vi "MCP2221_SetGpioSettings.vi"(8 "error in":errorcluster, 9 "handle in":i32, 10 "outputValues":u8[](array[numeric]), 11 "pinDirections":u8[](array[numeric])) -> (0 "error out":errorcluster, 1 "handle out":i32, 3 "return type":i32)   [LabVIEW 2025]
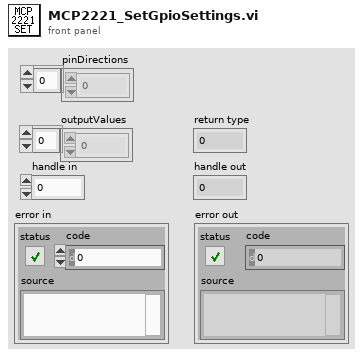
[diagram p1: front panel]
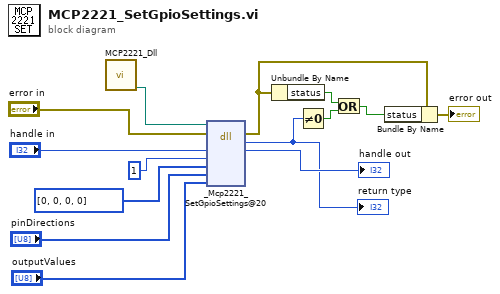
[diagram p0: block diagram]
diagram:
  n1 = call "MCP2221_Dll.vi"() -> ("dll path"=w8:path)  [unwired: 11 in]
  n2 = dll-call lib="?" fn="_Mcp2221_SetGpioSettings@20"(path in=w8, error in="error in", "handle"="handle in", "whichToSet"=u8 1, "pinFunctions"=u8[] [0, 0, 0, 0], "pinDirections"="pinDirections", "outputValues"="outputValues") -> (error out=w3:errorcluster, "return type"=w1:i32, "handle"=→"handle out":i32)  [unwired: 5 in, 1 out]
  "return type" <- w1
  n3 = Unbundle By Name(w3) -> ("status"=w6:bool)
  n4 = Not Equal To 0?(x=w1) -> (x != 0?=w2:bool)
  n5 = Or(x=w6, y=w2) -> (x .or. y?=w4:bool)
  n6 = Bundle By Name(cluster=w3, "status"=w4) -> (→"error out":errorcluster)
